vi "sub_strain-calmapping.vi"(11 "input":waveform(dbl)[](array[waveform])) -> (3 "output":waveform(dbl)[](array[waveform]))   [LabVIEW 2013]
panel:
  in  "sim":u8
  out "XY 그래프":cluster{dbl[], dbl[]}(graph)
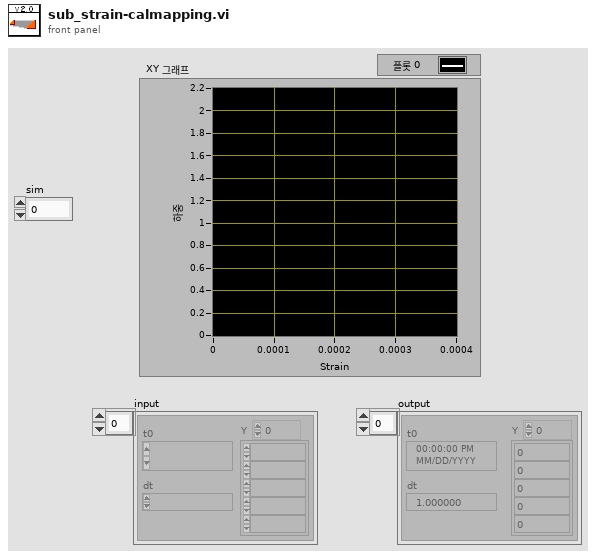
[diagram p1: front panel]
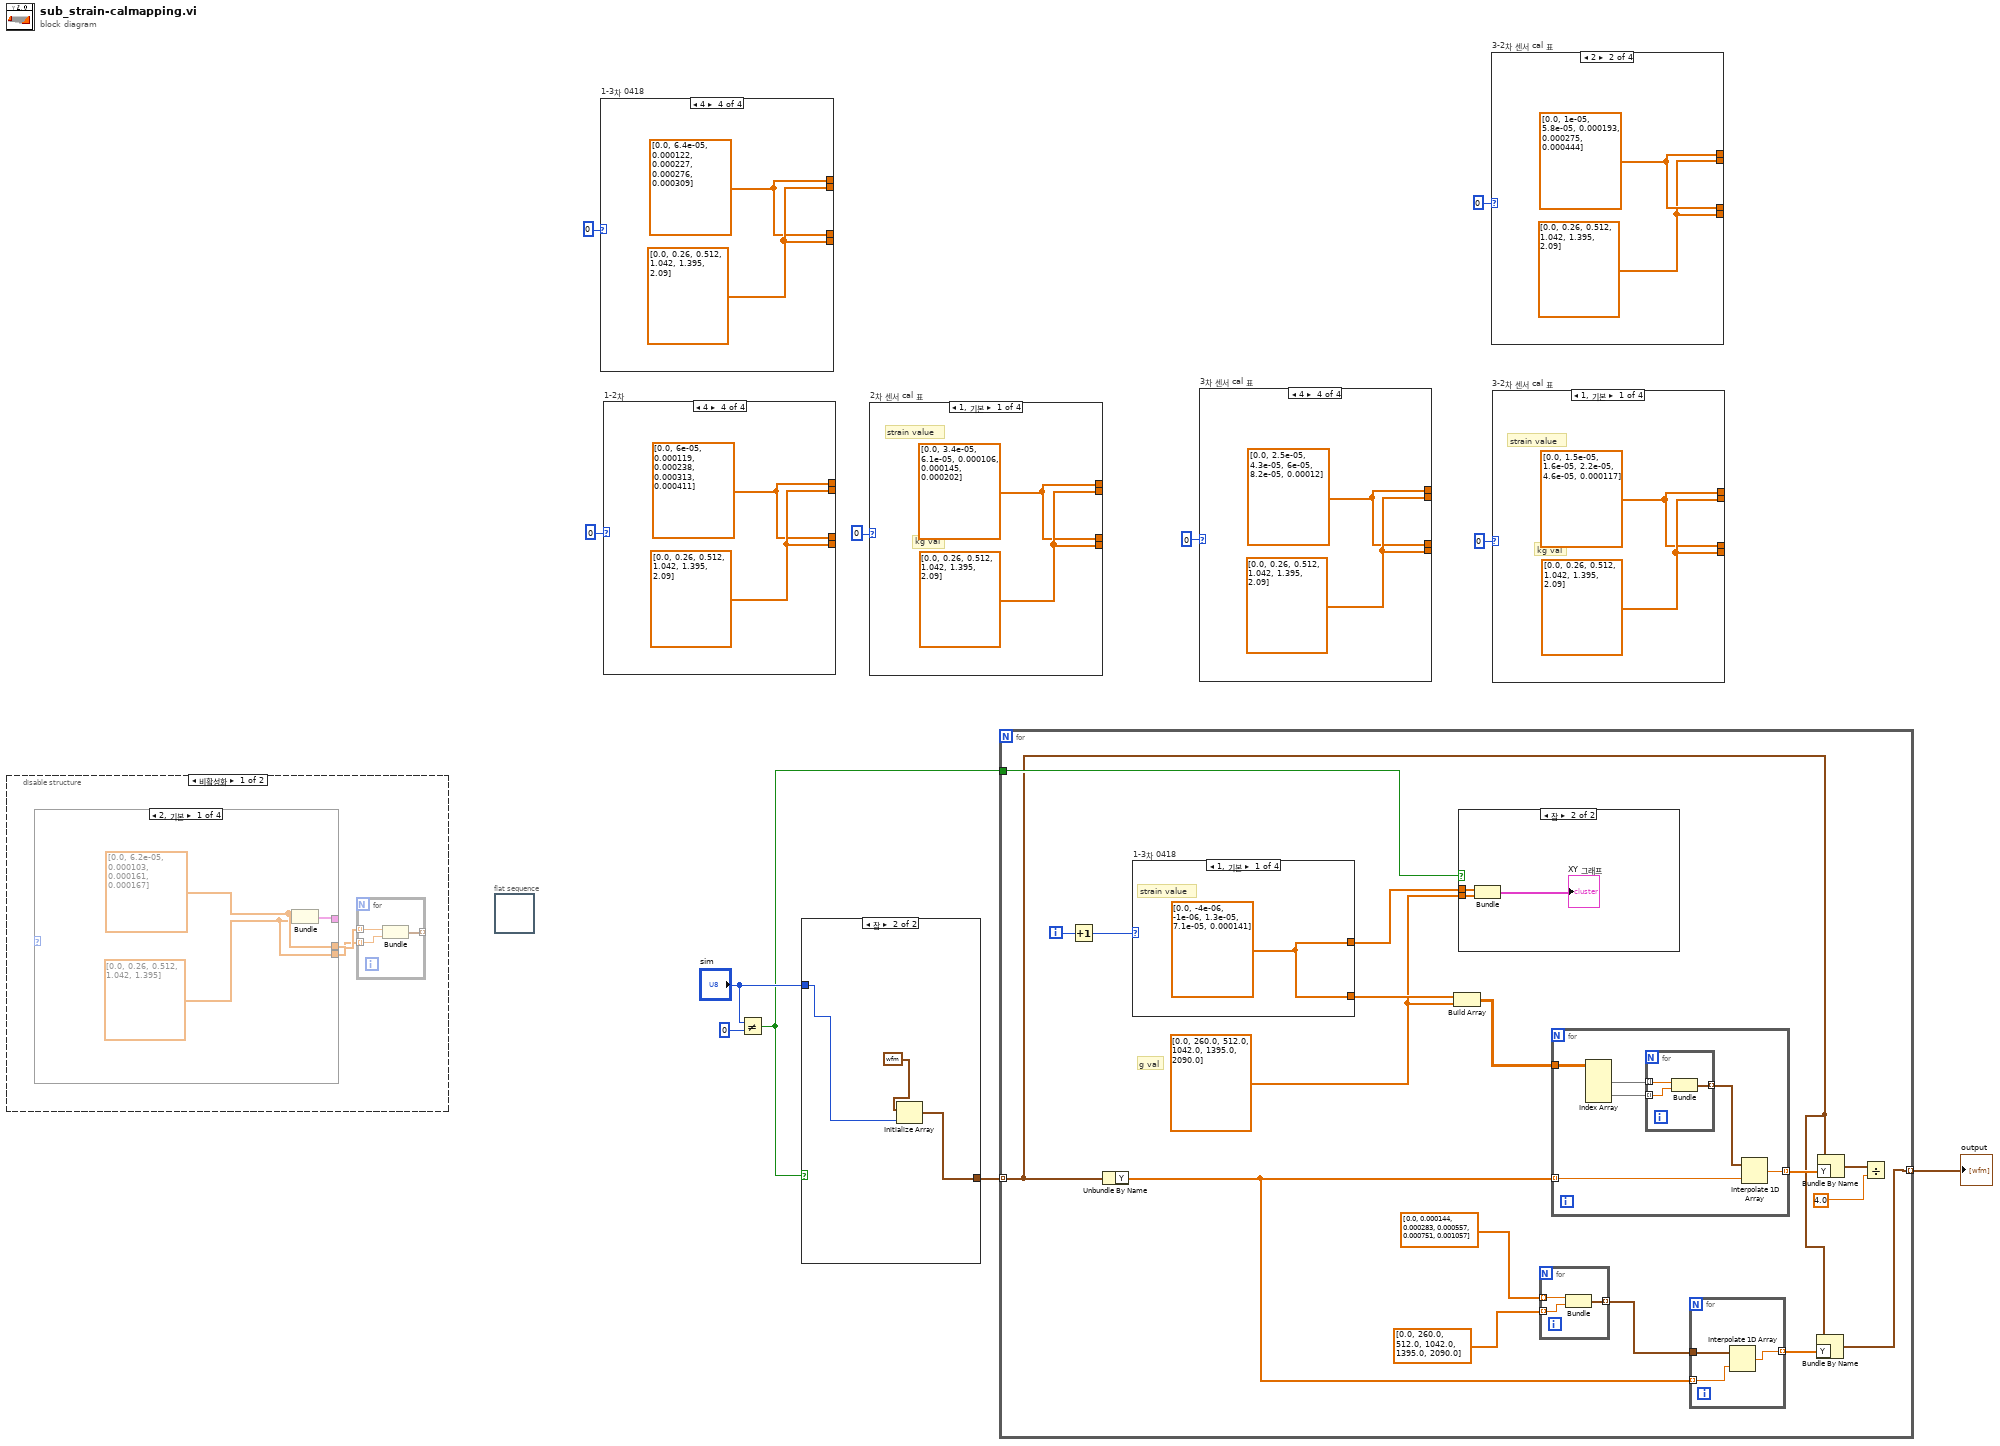
[diagram p0: block diagram]
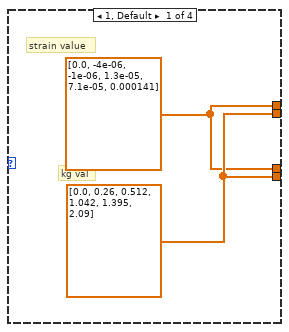
[diagram p2: hidden frame]
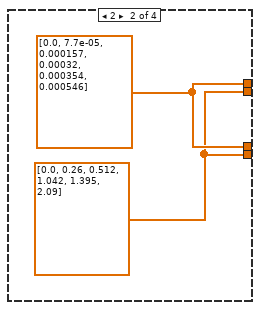
[diagram p3: hidden frame]
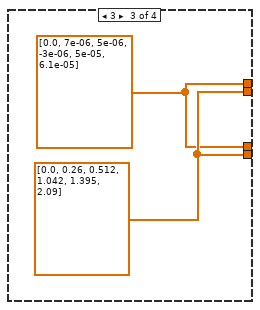
[diagram p4: hidden frame]
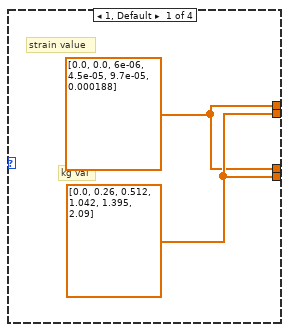
[diagram p5: hidden frame]
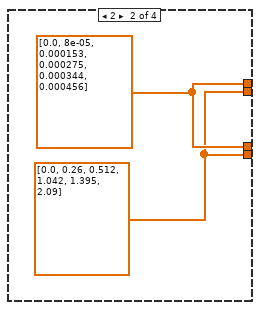
[diagram p6: hidden frame]
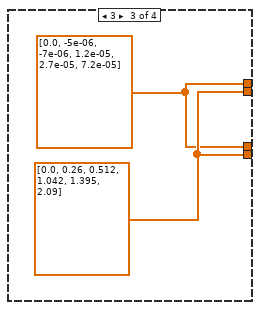
[diagram p7: hidden frame]
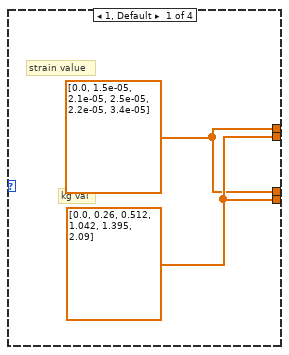
[diagram p8: hidden frame]
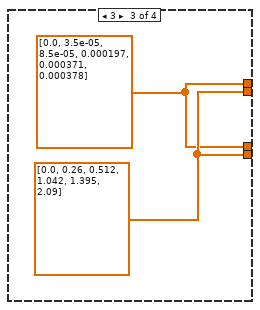
[diagram p9: hidden frame]
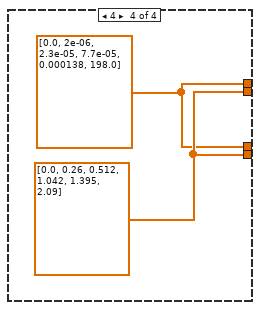
[diagram p10: hidden frame]
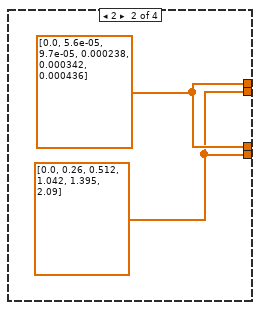
[diagram p11: hidden frame]
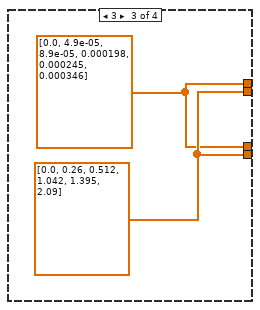
[diagram p12: hidden frame]
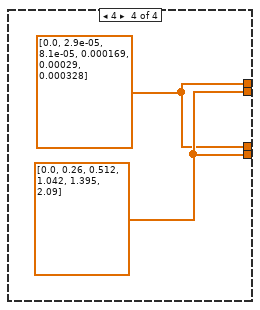
[diagram p13: hidden frame]
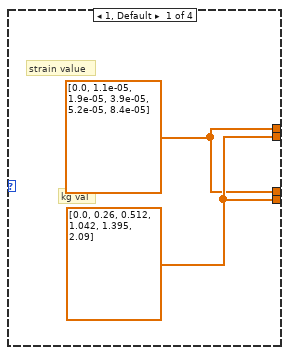
[diagram p14: hidden frame]
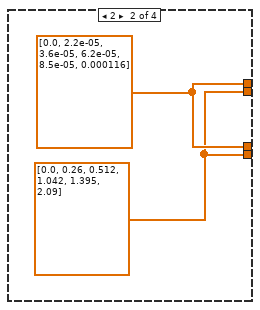
[diagram p15: hidden frame]
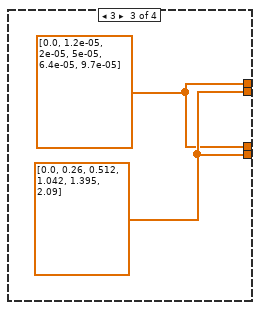
[diagram p16: hidden frame]
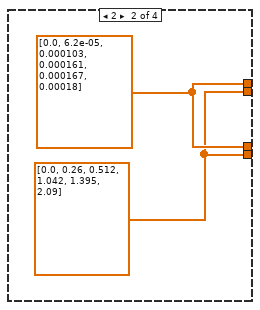
[diagram p17: hidden frame]
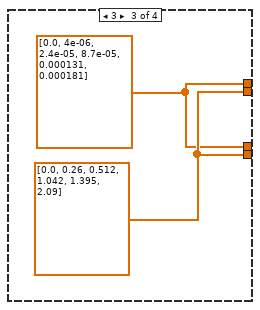
[diagram p18: hidden frame]
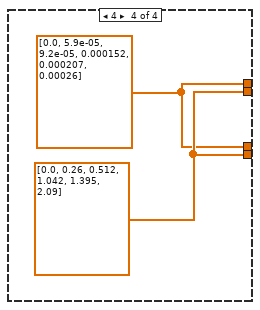
[diagram p19: hidden frame]
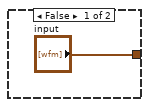
[diagram p20: hidden frame]
diagram:
  n1 = disable-structure shown="비활성화" {
    frame Disabled {
      n2 = case shown="2, 기본" {
        selector: _ -> [_ _ _ _]
        tunnel: [w19 w22 w25 w28] -> _
        tunnel: [w18 w21 w24 w27] -> w13
        tunnel: [w17 w20 w23 w26] -> w12
        frame 2, Default {
          w17 = dbl[] [0.0, 0.26, 0.512, 1.042, 1.395]
          w18 = dbl[] [0.0, 6.2e-05, 0.000103, 0.000161, 0.000167]
          n3 = Bundle(w18, w17) -> (w19:cluster{dbl[], dbl[]})  [unwired: 1 in]
        }
        frame 3 {
          w20 = dbl[] [0.0, 0.26, 0.512, 1.042, 1.395]
          w21 = dbl[] [0.0, 4e-06, 2.4e-05, 8.7e-05, 0.000131]
          n4 = Bundle(w21, w20) -> (w22:cluster{dbl[], dbl[]})  [unwired: 1 in]
        }
        frame 4 {
          w23 = dbl[] [0.0, 0.26, 0.512, 1.042, 1.395]
          w24 = dbl[] [0.0, 5.9e-05, 9.2e-05, 0.000152, 0.000207]
          n5 = Bundle(w24, w23) -> (w25:cluster{dbl[], dbl[]})  [unwired: 1 in]
        }
        frame 1 {
          w26 = dbl[] [0.0, 0.26, 0.512, 1.042, 1.395]
          w27 = dbl[] [0.0, 3.4e-05, 6.1e-05, 0.000106, 0.000145]
          n6 = Bundle(w27, w26) -> (w28:cluster{dbl[], dbl[]})  [unwired: 1 in]
        }
      }
      n7 = for {
        tunnel: w13 -> [w16] mode=indexing
        tunnel: w12 -> [w15] mode=indexing
        tunnel: [w14] -> _ mode=indexing
        n8 = Bundle(w16, w15) -> (w14:cluster{dbl, dbl})  [unwired: 1 in]
      }
    }
    frame Enabled {
    }
  }
  n9 = flat-sequence {
    frame #0 {
    }
  }
  n10 = case "1-3차 0418" shown="4" 0 {
    tunnel: [w29 w32 w33 w35] -> _
    tunnel: [w30 w31 w34 w36] -> _
    tunnel: [w29 w32 w33 w35] -> _
    tunnel: [w30 w31 w34 w36] -> _
    frame 1, Default {
      w30 = dbl[] [0.0, 0.26, 0.512, 1.042, 1.395, 2.09]
      w29 = dbl[] [0.0, -4e-06, -1e-06, 1.3e-05, 7.1e-05, 0.000141]
      # "kg val"
      # "strain value"
    }
    frame 2 {
      w31 = dbl[] [0.0, 0.26, 0.512, 1.042, 1.395, 2.09]
      w32 = dbl[] [0.0, 7.7e-05, 0.000157, 0.00032, 0.000354, 0.000546]
    }
    frame 3 {
      w34 = dbl[] [0.0, 0.26, 0.512, 1.042, 1.395, 2.09]
      w33 = dbl[] [0.0, 7e-06, 5e-06, -3e-06, 5e-05, 6.1e-05]
    }
    frame 4 {
      w36 = dbl[] [0.0, 0.26, 0.512, 1.042, 1.395, 2.09]
      w35 = dbl[] [0.0, 6.4e-05, 0.000122, 0.000227, 0.000276, 0.000309]
    }
  }
  n11 = case "1-2차" shown="4" 0 {
    tunnel: [w37 w40 w41 w43] -> _
    tunnel: [w38 w39 w42 w44] -> _
    tunnel: [w37 w40 w41 w43] -> _
    tunnel: [w38 w39 w42 w44] -> _
    frame 1, Default {
      w38 = dbl[] [0.0, 0.26, 0.512, 1.042, 1.395, 2.09]
      w37 = dbl[] [0.0, 0.0, 6e-06, 4.5e-05, 9.7e-05, 0.000188]
      # "kg val"
      # "strain value"
    }
    frame 2 {
      w39 = dbl[] [0.0, 0.26, 0.512, 1.042, 1.395, 2.09]
      w40 = dbl[] [0.0, 8e-05, 0.000153, 0.000275, 0.000344, 0.000456]
    }
    frame 3 {
      w42 = dbl[] [0.0, 0.26, 0.512, 1.042, 1.395, 2.09]
      w41 = dbl[] [0.0, -5e-06, -7e-06, 1.2e-05, 2.7e-05, 7.2e-05]
    }
    frame 4 {
      w44 = dbl[] [0.0, 0.26, 0.512, 1.042, 1.395, 2.09]
      w43 = dbl[] [0.0, 6e-05, 0.000119, 0.000238, 0.000313, 0.000411]
    }
  }
  n12 = Not Equal?(x="sim", y=u8 0) -> (x != y?=w7:bool)
  n13 = case shown="참" w7 {
    tunnel: ["input" w46] -> w11
    tunnel: "sim" -> [_ w47]
    frame False {
    }
    frame True {
      n14 = Initialize Array(waveform(dbl) {"t0"=timestamp(0 s since 1904-01-01), "dt"=0.0, "Y"=[]} ("waveform"), w47) -> (w46:waveform(dbl)[])
    }
  }
  n15 = case "2차 센서 cal 표" shown="1, 기본" 0 {
    tunnel: [w49 w52 w53 w55] -> _
    tunnel: [w50 w51 w54 w56] -> _
    tunnel: [w49 w52 w53 w55] -> _
    tunnel: [w50 w51 w54 w56] -> _
    frame 1, Default {
      w50 = dbl[] [0.0, 0.26, 0.512, 1.042, 1.395, 2.09]
      w49 = dbl[] [0.0, 3.4e-05, 6.1e-05, 0.000106, 0.000145, 0.000202]
      # "kg val"
      # "strain value"
    }
    frame 2 {
      w51 = dbl[] [0.0, 0.26, 0.512, 1.042, 1.395, 2.09]
      w52 = dbl[] [0.0, 6.2e-05, 0.000103, 0.000161, 0.000167, 0.00018]
    }
    frame 3 {
      w54 = dbl[] [0.0, 0.26, 0.512, 1.042, 1.395, 2.09]
      w53 = dbl[] [0.0, 4e-06, 2.4e-05, 8.7e-05, 0.000131, 0.000181]
    }
    frame 4 {
      w56 = dbl[] [0.0, 0.26, 0.512, 1.042, 1.395, 2.09]
      w55 = dbl[] [0.0, 5.9e-05, 9.2e-05, 0.000152, 0.000207, 0.00026]
    }
  }
  n16 = for {
    tunnel: w11 -> [w59] mode=indexing
    tunnel: [w57] -> w10 mode=indexing
    tunnel: w7 -> [w68]
    i -> [w69]
    w64 = dbl[] [0.0, 260.0, 512.0, 1042.0, 1395.0, 2090.0]
    # "g val"
    n17 = Increment(x=w69) -> (x+1=w67:i32)
    n18 = Unbundle By Name(w59) -> ("Y"=w60:dbl[])
    n19 = case "1-3차 0418" shown="1, 기본" w67 {
      tunnel: [w80 w81 w82 w83] -> w65
      tunnel: [w80 w81 w82 w83] -> w66
      frame 1, Default {
        w80 = dbl[] [0.0, -4e-06, -1e-06, 1.3e-05, 7.1e-05, 0.000141]
        # "strain value"
      }
      frame 2 {
        w81 = dbl[] [0.0, 7.7e-05, 0.000157, 0.00032, 0.000354, 0.000546]
      }
      frame 3 {
        w82 = dbl[] [0.0, 7e-06, 5e-06, -3e-06, 5e-05, 6.1e-05]
      }
      frame 4 {
        w83 = dbl[] [0.0, 6.4e-05, 0.000122, 0.000227, 0.000276, 0.000309]
      }
    }
    n20 = Build Array(w65, w64) -> (w72:dbl[][])
    n21 = case shown="참" w68 {
      tunnel: w64 -> [_ w85]
      tunnel: w66 -> [_ w84]
      frame False {
      }
      frame True {
        n22 = Bundle(w84, w85) -> (→"XY 그래프":cluster{dbl[], dbl[]})  [unwired: 1 in]
      }
    }
    n23 = for {
      tunnel: dbl[] [0.0, 0.000144, 0.000283, 0.000557, 0.000751, 0.001057] ("x") -> [w79] mode=indexing
      tunnel: dbl[] [0.0, 260.0, 512.0, 1042.0, 1395.0, 2090.0] ("y") -> [w78] mode=indexing
      tunnel: [w77] -> w61 mode=indexing
      n24 = Bundle(w79, w78) -> (w77:cluster{dbl, dbl})  [unwired: 1 in]
    }
    n25 = for {
      tunnel: w72 -> [w88]
      tunnel: [w90] -> w73 mode=indexing
      tunnel: w60 -> [w89] mode=indexing
      n26 = Index Array(array=w88) -> (element #1=w92:dbl[], element #2=w91:dbl[])  [unwired: 4 in]
      n27 = for {
        tunnel: w92 -> [w95] mode=indexing
        tunnel: w91 -> [w94] mode=indexing
        tunnel: [w93] -> w87 mode=indexing
        n28 = Bundle(w95, w94) -> (w93:cluster{dbl, dbl})  [unwired: 1 in]
      }
      n29 = Interpolate 1D Array(1:w89, 2:w87) -> (0:w90:dbl)
    }
    n30 = for {
      tunnel: w61 -> [w76]
      tunnel: w60 -> [w75] mode=indexing
      tunnel: [w74] -> w58 mode=indexing
      n31 = Interpolate 1D Array(1:w75, 2:w76) -> (0:w74:dbl)
    }
    n32 = Bundle By Name(cluster=w59, "Y"=w58) -> (w57:waveform(dbl))
    n33 = Bundle By Name(cluster=w59, "Y"=w73) -> (w70:waveform(dbl))
    n34 = Divide(x=w70, y=4.0) -> ()  [unwired: 1 out]
  }
  "output" <- w10
  n35 = case "3차 센서 cal 표" shown="4" 0 {
    tunnel: [w96 w99 w100 w102] -> _
    tunnel: [w97 w98 w101 w103] -> _
    tunnel: [w96 w99 w100 w102] -> _
    tunnel: [w97 w98 w101 w103] -> _
    frame 1, Default {
      w97 = dbl[] [0.0, 0.26, 0.512, 1.042, 1.395, 2.09]
      w96 = dbl[] [0.0, 1.1e-05, 1.9e-05, 3.9e-05, 5.2e-05, 8.4e-05]
      # "kg val"
      # "strain value"
    }
    frame 2 {
      w98 = dbl[] [0.0, 0.26, 0.512, 1.042, 1.395, 2.09]
      w99 = dbl[] [0.0, 2.2e-05, 3.6e-05, 6.2e-05, 8.5e-05, 0.000116]
    }
    frame 3 {
      w101 = dbl[] [0.0, 0.26, 0.512, 1.042, 1.395, 2.09]
      w100 = dbl[] [0.0, 1.2e-05, 2e-05, 5e-05, 6.4e-05, 9.7e-05]
    }
    frame 4 {
      w103 = dbl[] [0.0, 0.26, 0.512, 1.042, 1.395, 2.09]
      w102 = dbl[] [0.0, 2.5e-05, 4.3e-05, 6e-05, 8.2e-05, 0.00012]
    }
  }
  n36 = case "3-2차 센서 cal 표" shown="2" 0 {
    tunnel: [w104 w107 w108 w110] -> _
    tunnel: [w105 w106 w109 w111] -> _
    tunnel: [w104 w107 w108 w110] -> _
    tunnel: [w105 w106 w109 w111] -> _
    frame 1, Default {
      w105 = dbl[] [0.0, 0.26, 0.512, 1.042, 1.395, 2.09]
      w104 = dbl[] [0.0, 1.5e-05, 2.1e-05, 2.5e-05, 2.2e-05, 3.4e-05]
      # "kg val"
      # "strain value"
    }
    frame 2 {
      w106 = dbl[] [0.0, 0.26, 0.512, 1.042, 1.395, 2.09]
      w107 = dbl[] [0.0, 1e-05, 5.8e-05, 0.000193, 0.000275, 0.000444]
    }
    frame 3 {
      w109 = dbl[] [0.0, 0.26, 0.512, 1.042, 1.395, 2.09]
      w108 = dbl[] [0.0, 3.5e-05, 8.5e-05, 0.000197, 0.000371, 0.000378]
    }
    frame 4 {
      w111 = dbl[] [0.0, 0.26, 0.512, 1.042, 1.395, 2.09]
      w110 = dbl[] [0.0, 2e-06, 2.3e-05, 7.7e-05, 0.000138, 198.0]
    }
  }
  n37 = case "3-2차 센서 cal 표" shown="1, 기본" 0 {
    tunnel: [w112 w115 w116 w118] -> _
    tunnel: [w113 w114 w117 w119] -> _
    tunnel: [w112 w115 w116 w118] -> _
    tunnel: [w113 w114 w117 w119] -> _
    frame 1, Default {
      w113 = dbl[] [0.0, 0.26, 0.512, 1.042, 1.395, 2.09]
      w112 = dbl[] [0.0, 1.5e-05, 1.6e-05, 2.2e-05, 4.6e-05, 0.000117]
      # "kg val"
      # "strain value"
    }
    frame 2 {
      w114 = dbl[] [0.0, 0.26, 0.512, 1.042, 1.395, 2.09]
      w115 = dbl[] [0.0, 5.6e-05, 9.7e-05, 0.000238, 0.000342, 0.000436]
    }
    frame 3 {
      w117 = dbl[] [0.0, 0.26, 0.512, 1.042, 1.395, 2.09]
      w116 = dbl[] [0.0, 4.9e-05, 8.9e-05, 0.000198, 0.000245, 0.000346]
    }
    frame 4 {
      w119 = dbl[] [0.0, 0.26, 0.512, 1.042, 1.395, 2.09]
      w118 = dbl[] [0.0, 2.9e-05, 8.1e-05, 0.000169, 0.00029, 0.000328]
    }
  }
